vi "oa_Get Angular Speed (1 Tach).vi"(7 "reset? (True)":bool=TRUE, 8 "error in (no error)":errorcluster, 9 "input data duration [s]":dbl format="%0.2f", 10 "pulse/revolution (1)":i32=1, 11 "pulse positions [s]":dbl[](array[numeric]) format="%.2f") -> (0 "error out":errorcluster, 1 "no tacho? (F)":bool, 2 "pulse positions [s]":dbl[](array[numeric]) format="%.2f", 3 "speed profile":T1 {"speed [RPM]" format="%.2f"; "time [s]" format="%.2f"})   [LabVIEW 2017, in "SoundVib_TachProcess.lvlib"]
doc: "Computes the angular speed at each pulse edge contained in <B>pulse positions [s]</B>."
uses:
  <vilib>/addons/Sound and Vibration/Order Analysis/Tach Process/SoundVib_TachProcess.lvlib
  <vilib>/addons/Sound and Vibration/Order Analysis/Tach Process/SubVIs/speed profile.ctl
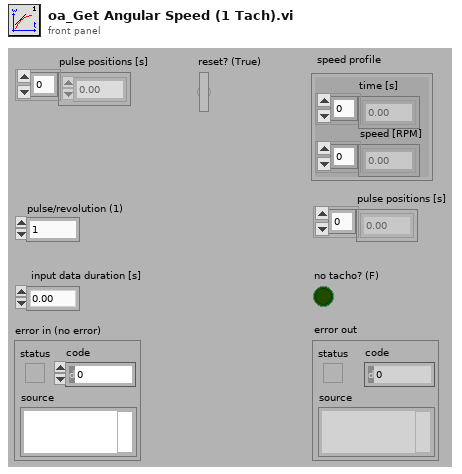
[diagram p1: front panel]
types:
  T1 = typedef "SoundVib_TachProcess.lvlib/speed profile.ctl" = cluster{"time [s]":dbl[], "speed [RPM]":dbl[]}
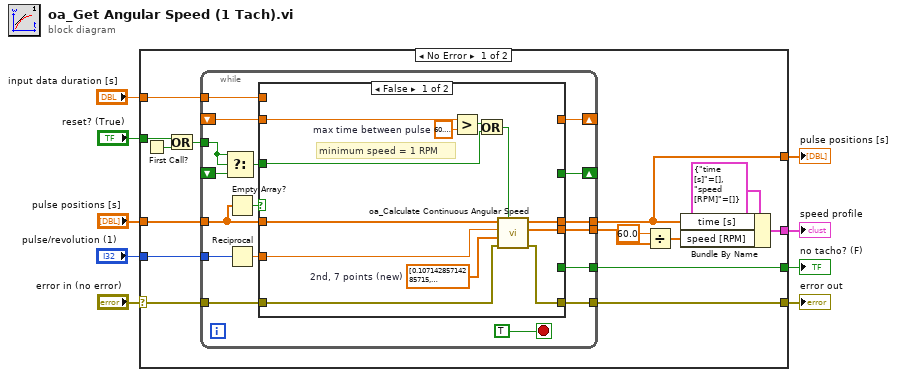
[diagram p0: block diagram]
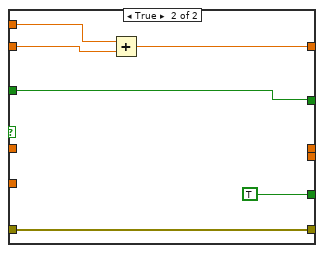
[diagram p2: hidden frame]
diagram:
  n1 = case shown="No Error" "error in (no error)" {
    selector: "error in (no error)" -> [w18 w60]
    tunnel: "pulse positions [s]" -> [w23 _]
    tunnel: [w22 _] -> w8
    tunnel: "pulse/revolution (1)" -> [w13 _]
    tunnel: [w17 w60] -> w6
    tunnel: [w16 _] -> w4
    tunnel: [w19 _] -> w3
    tunnel: "input data duration [s]" -> [w15 _]
    tunnel: "reset? (True)" -> [w11 _]
    frame No Error {
      n2 = First Call?() -> (First Call?: T/F=w12:bool)
      n3 = Or(x=w11, y=w12) -> (x .or. y?=w10:bool)
      n4 = while {
        tunnel: w23 -> [w27]
        tunnel: [w41] -> w20
        tunnel: w10 -> [w32]
        tunnel: [w40] -> w19
        tunnel: w18 -> [w39]
        tunnel: [w38] -> w17
        tunnel: [w37] -> w16
        shift-right: [w33] -> _
        shift-left: _ -> [w34]
        tunnel: w15 -> [w35]
        shift-right: [w29] -> _
        shift-left: _ -> [w31]
        tunnel: w13 -> [w26]
        stop <- TRUE stop-if-true
        n5 = Select(t=w32, s=w32, f=w31) -> (s? t:f=w30:bool)
        n6 = Empty Array?(array=w27) -> (empty?=w28:bool)
        n7 = Reciprocal(x=w26) -> (1/x=w25:dbl)
        n8 = case shown="False" w28 {
          tunnel: w27 -> [w43 _]
          tunnel: w25 -> [w50 _]
          tunnel: [w53 w59] -> w38
          tunnel: [w52 _] -> w41
          tunnel: [w51 _] -> w40
          tunnel: w39 -> [w49 w59]
          tunnel: [_ TRUE] -> w37
          tunnel: w35 -> [_ w57]
          tunnel: w34 -> [w47 w56]
          tunnel: [_ w55] -> w33
          tunnel: w30 -> [w42 w54]
          tunnel: [_ w54] -> w29
          frame False {
            w46 = 60.499  # max time between pulse
            w48 = dbl[] [0.10714285714285715, 0.07142857142857142, 0.035714285714285705, -1.5209319782164736e-17, -0.03571428571428571, -0.07142857142857142, -0.10714285714285715]  # 2nd, 7 points (new)
            # "minimum speed = 1 RPM"
            n9 = Greater?(x=w47, y=w46) -> (0:w45:bool)
            n10 = Or(x=w45, y=w42) -> (x .or. y?=w44:bool)
            n11 = call <vilib>:"oa_Calculate Continuous Angular Speed.vi"("reset? (True)"=w44, "error in (no error)"=w49, "filter coefficients"=w48, "deltaX"=w50, "Y[n]"=w43) -> ("error out"=w53:errorcluster, "dY/dX[n]"=w52:dbl[], "pulse out"=w51:dbl[])  [unwired: 4 in]
          }
          frame True {
            n12 = Add(x=w57, y=w56) -> (x+y=w55:dbl)
          }
        }
      }
      n13 = Divide(x=60.0, y=w20) -> (x/y=w21:dbl[])
      n14 = Bundle By Name(cluster=T1 {"time [s]"=[], "speed [RPM]"=[]} ("speed profile"), "time [s]"=w19, "speed [RPM]"=w21) -> (w22:T1)
    }
    frame Error {
    }
  }
  "speed profile" <- w8
  "error out" <- w6
  "no tacho? (F)" <- w4
  "pulse positions [s]" <- w3
